vi "Base Error Code.vi"() -> (3 "base error code":i32)   [LabVIEW 2023, in "UDPlog.lvlib" / "UDPlog Transceiver.lvclass"]
uses:
  UDPlog Transceiver.lvclass
  UDPlog Transceiver.lvclass/UDPlog Transceiver.ctl
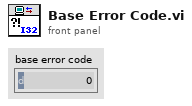
[diagram p1: front panel]
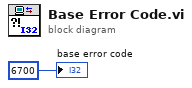
[diagram p0: block diagram]
diagram:
  "base error code" <- 6700 ("base error code")
